vi "Check Status (No Objects) - Wavelength meter.vi"(8 "error in (no error)":errorcluster, 11 "Cluster In":T3={"Exp Range Min"=0, "Exp Range Max"=0, "exposure mode"=enum."manual", "operation (meas. mode)"=enum."Measurement mode", "Exposure (ms)"=0, "Quiet Errors?"=FALSE, "Error Status"={"status"=FALSE, "code"=0, "source"=""}}) -> (0 "error out":errorcluster, 1 "Status":string, 2 "Ready?":bool, 3 "Cluster Out":T3={"Exp Range Min"=0, "Exp Range Max"=0, "exposure mode"=enum."manual", "operation (meas. mode)"=enum."Measurement mode", "Exposure (ms)"=0, "Quiet Errors?"=FALSE, "Error Status"={"status"=FALSE, "code"=0, "source"=""}})   [LabVIEW 2012]
doc: "(Dynamic) Check if the instrument is powered on and update its member fields with the instrument's current status. Optionally return a text status message."
uses:
  HighFinesse WS5/Variable Typedefs.llb/Exposure Mode.ctl
  HighFinesse WS5/Control typedefs.llb/Measurement Mode.ctl
  HighFinesse WS5/HighFinesse WS5.lvlib
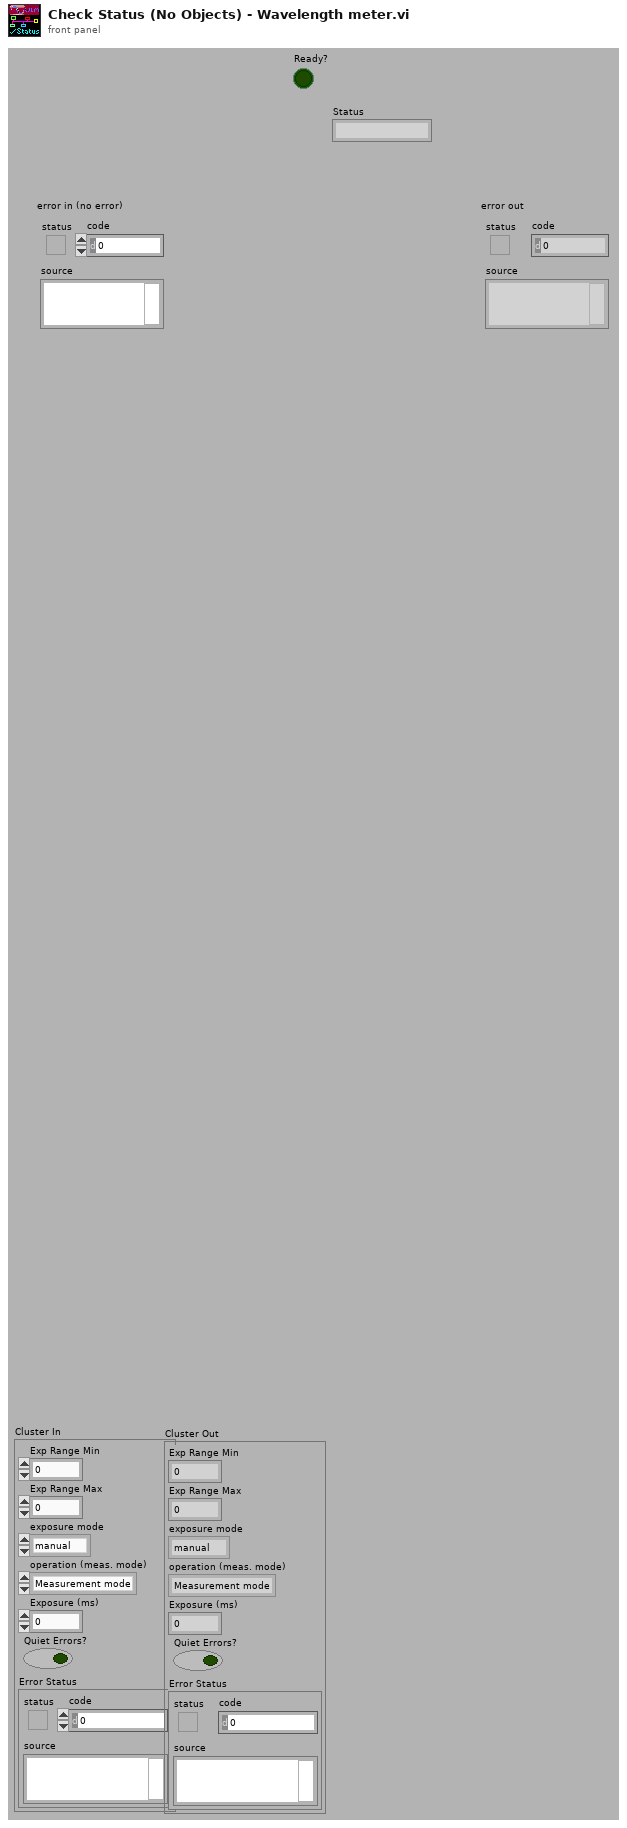
[diagram p1: front panel]
types:
  T1 = typedef "HighFinesse WS5.lvlib/Exposure Mode.ctl" = enum16{"manual", "automatic"}
  T2 = typedef "HighFinesse WS5.lvlib/Measurement Mode.ctl" = enum16{"Measurement off", "Adjustment mode", "Measurement mode"}
  T3 = cluster{"Exp Range Min":u32, "Exp Range Max":u32, "exposure mode":T1, "operation (meas. mode)":T2, "Exposure (ms)":u16, "Quiet Errors?":bool, "Error Status":errorcluster}
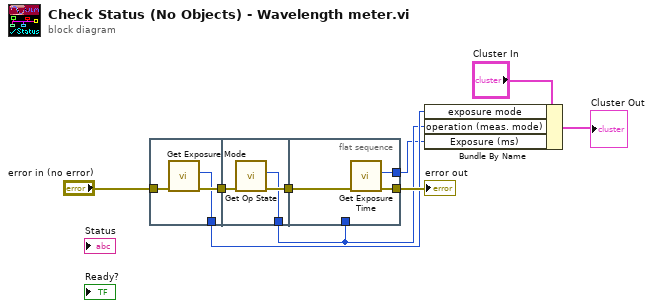
[diagram p0: block diagram]
diagram:
  n1 = flat-sequence {
    tunnel: "error in (no error)" -> [w12]
    tunnel: [w11] -> w9
    tunnel: [w10] -> w7
    tunnel: w9 -> [w15]
    tunnel: [w14] -> w6
    tunnel: [w13] -> w5
    tunnel: w5 -> [_]
    tunnel: [w17] -> w8
    tunnel: w6 -> [w18]
    tunnel: [w16] -> w4
    frame #0 {
      n2 = call "Get Exposure Mode.vi"("error in (no error)"=w12) -> ("error out"=w11:errorcluster, "exposure mode"=w10:T1)  [unwired: 9 in]
    }
    frame #1 {
      n3 = call "Get Op State.vi"("error in (no error)"=w15) -> ("error out"=w14:errorcluster, "operation (meas. mode)"=w13:T2)  [unwired: 9 in]
    }
    frame #2 {
      n4 = call "Get Exposure Time.vi"("error in (no error)"=w18) -> ("error out"=w17:errorcluster, "Exposure (ms)"=w16:u16)  [unwired: 9 in]
    }
  }
  n5 = Bundle By Name(cluster="Cluster In", "exposure mode"=w7, "operation (meas. mode)"=w5, "Exposure (ms)"=w4) -> (→"Cluster Out":T3)
  "error out" <- w8
